vi "Configrue AUX Port.vi"(6 "Output Sample Clock Polarity (0: Positive)":i32(ring) items=["Positive", "Negative"], 7 "Operating Mode (0: Dedicated)":i32(ring) items=["Dedicated", "Multiplexed"], 8 "error in (no error)":errorcluster, 9 "Input Strobe Polarity (0: Positive)":i32(ring) items=["Positive", "Negative"], 10 "Data Input Mode (0: Free)":i32(ring) items=["Free", "User"], 11 "VISA resource name":refnum<visa-resource-name>) -> (0 "error out":errorcluster, 3 "VISA resource name out":refnum<visa-resource-name>)   [LabVIEW 2014, in "Agilent PSG MXG Series.lvlib"]
doc: "Configures AUX port settings.\n\n<B>Notes:</B>\n(1) This VI is valid only in N5172B and N5182B that install <B>Option 660</B>."
uses:
  Agilent PSG MXG Series.lvlib
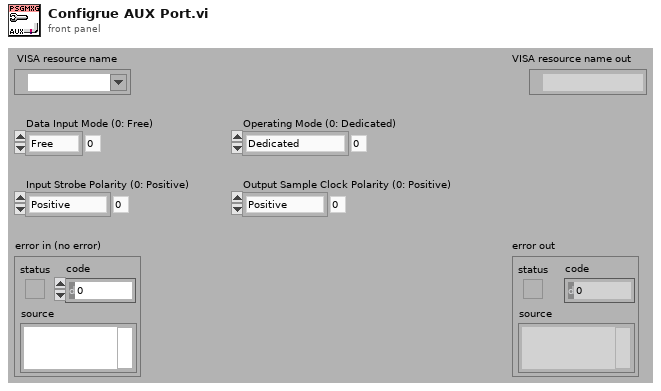
[diagram p1: front panel]
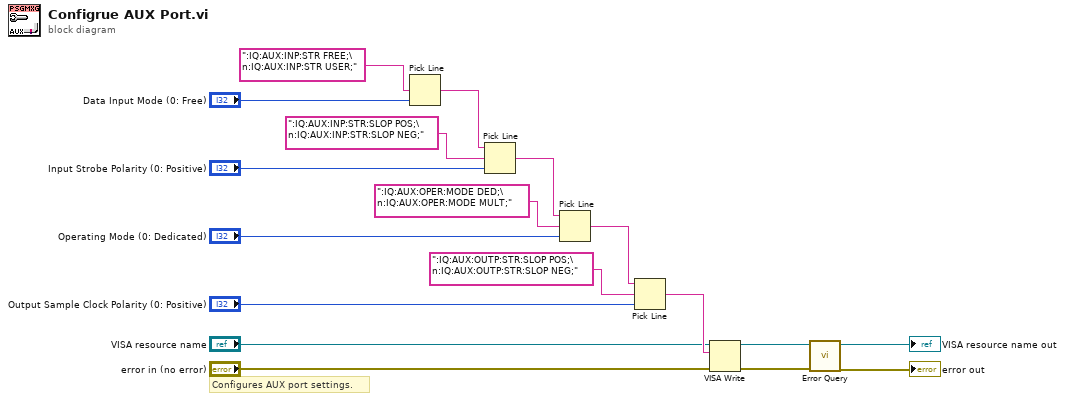
[diagram p0: block diagram]
diagram:
  # "Configures AUX port settings."
  n1 = Pick Line(multi-line string=":IQ:AUX:INP:STR FREE;\n:IQ:AUX:INP:STR USER;", line index="Data Input Mode (0: Free)") -> (output string=w14:string)  [unwired: 1 out]
  n2 = Pick Line(string ("")=w14, multi-line string=":IQ:AUX:INP:STR:SLOP POS;\n:IQ:AUX:INP:STR:SLOP NEG;", line index="Input Strobe Polarity (0: Positive)") -> (output string=w11:string)
  n3 = Pick Line(string ("")=w11, multi-line string=":IQ:AUX:OPER:MODE DED;\n:IQ:AUX:OPER:MODE MULT;", line index="Operating Mode (0: Dedicated)") -> (output string=w8:string)
  n4 = Pick Line(string ("")=w8, multi-line string=":IQ:AUX:OUTP:STR:SLOP POS;\n:IQ:AUX:OUTP:STR:SLOP NEG;", line index="Output Sample Clock Polarity (0: Positive)") -> (output string=w7:string)
  n5 = VISA Write(VISA resource name="VISA resource name", write buffer=w7, error in (no error)="error in (no error)") -> (VISA resource name out=w4:refnum<visa-resource-name>, error out=w3:errorcluster)  [unwired: 1 out]
  n6 = call "Error Query.vi"("error in (no error)"=w3, "VISA resource name"=w4) -> ("error out"=→"error out":errorcluster, "VISA resource name out"=→"VISA resource name out":refnum<visa-resource-name>)  [unwired: 8 out]
